vi "Dark_Current_Initialization_Sub_VI.vi"(7 "VISA resource name 2":refnum<visa-resource-name>, 11 "Channel #":i32) -> (0 "error out":errorcluster, 1 "BoardHandle out":T1, 3 "Channel # 2":i32)   [LabVIEW 2018]
uses:
  Program Files (x86)/National Instruments/LabVIEW 2020/instr.lib/CAEN PSM/CAEN PSM.lvlib
panel:
  in  "VISA resource name":refnum<visa-resource-name>
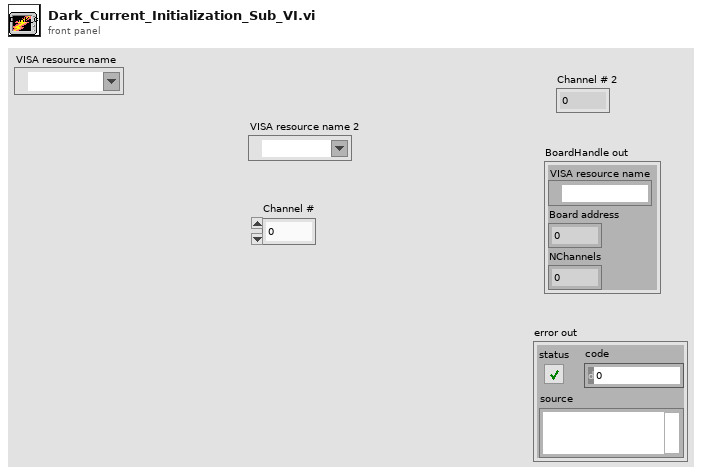
[diagram p1: front panel]
types:
  T1 = cluster{"VISA resource name":refnum<visa-resource-name>, "Board address":u8, "NChannels":u8}
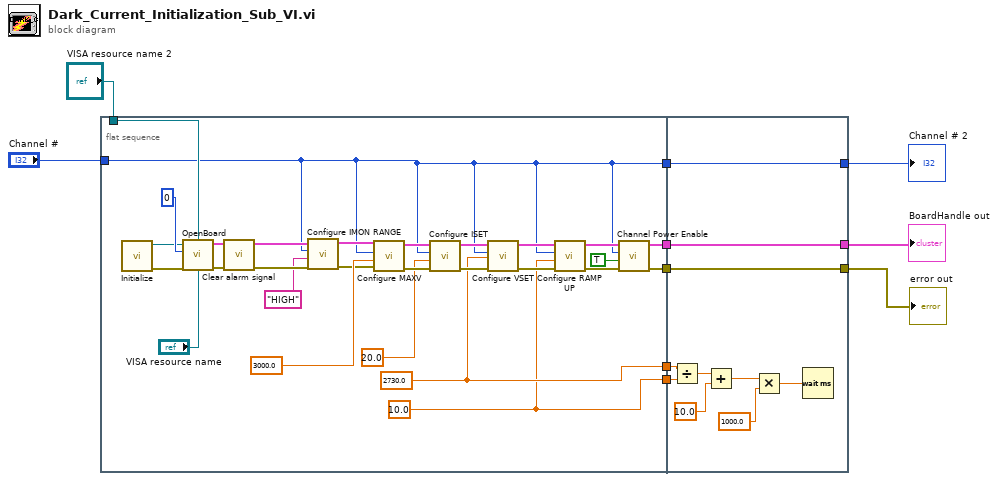
[diagram p0: block diagram]
diagram:
  n1 = flat-sequence {
    tunnel: [w22] -> w10
    tunnel: [w21] -> w9
    tunnel: ["VISA resource name"] -> _
    tunnel: [w20] -> w8
    tunnel: [w19] -> w7
    tunnel: [w11] -> w6
    tunnel: "Channel #" -> [w11]
    tunnel: "VISA resource name 2" -> [_]
    tunnel: w10 -> [w42]
    tunnel: w9 -> [w41]
    tunnel: [w38] -> w3
    tunnel: w8 -> [w38]
    tunnel: [w40] -> w4
    tunnel: w7 -> [w40]
    tunnel: [w39] -> w2
    tunnel: w6 -> [w39]
    frame #0 {
      w22 = 2730.0 ("Voltage Set (Volts)")
      w21 = 10.0 ("Voltage Ramp Up (V/s)")
      n2 = call "Initialize.vi"("VISA resource name"="VISA resource name") -> ("error out"=w32:errorcluster, "VISA resource name out"=w28:refnum<visa-resource-name>)  [unwired: 9 in]
      n3 = call "OpenBoard.vi"("error in (no error)"=w32, "Board Address"=0, "VISA resource name"=w28) -> ("error out"=w33:errorcluster, "BoardHandle"=w27:T1)  [unwired: 7 in]
      n4 = call "Clear alarm signal.vi"("error in (no error)"=w33, "BoardHandle"=w27) -> ("error out"=w17:errorcluster, "BoardHandle out"=w16:T1)  [unwired: 8 in]
      n5 = call "Configure IMON RANGE.vi"("error in (no error)"=w17, "IMon range (LOW)"="HIGH", "Channel (0)"=w11, "BoardHandle"=w16) -> ("error out"=w13:errorcluster, "BoardHandle out"=w14:T1)  [unwired: 6 in]
      n6 = call "Configure MAXV.vi"("error in (no error)"=w13, "Voltage Max (0.0 V)"=3000.0 ("VMax (Volts)"), "Channel (0)"=w11, "BoardHandle"=w14) -> ("error out"=w34:errorcluster, "BoardHandle out"=w26:T1)  [unwired: 6 in]
      n7 = call "Configure ISET.vi"("error in (no error)"=w34, "Current Limit (0.00 uA)"=20.0 ("Current Limit (uA)"), "Channel (0)"=w11, "BoardHandle"=w26) -> ("error out"=w35:errorcluster, "BoardHandle out"=w25:T1)  [unwired: 6 in]
      n8 = call "Configure VSET.vi"("error in (no error)"=w35, "Voltage Level (0.0 V)"=w22, "Channel (0)"=w11, "BoardHandle"=w25) -> ("error out"=w36:errorcluster, "BoardHandle out"=w24:T1)  [unwired: 6 in]
      n9 = call "Configure RAMP UP.vi"("error in (no error)"=w36, "Voltage ramp up (0 V/s)"=w21, "Channel (0)"=w11, "BoardHandle"=w24) -> ("error out"=w37:errorcluster, "BoardHandle out"=w23:T1)  [unwired: 6 in]
      n10 = call "Channel Power Enable.vi"("error in (no error)"=w37, "Enable (OFF)"=TRUE ("Boolean"), "Channel (0)"=w11, "BoardHandle"=w23) -> ("error out"=w19:errorcluster, "BoardHandle out"=w20:T1)  [unwired: 6 in]
    }
    frame #1 {
      n11 = Divide(x=w42, y=w41) -> (x/y=w45:dbl)
      n12 = Add(x=w45, y=10.0) -> (x+y=w46:dbl)
      n13 = Multiply(x=w46, y=1000.0) -> (x*y=w47:dbl)
      n14 = Wait (ms)(milliseconds to wait=w47) -> ()  [unwired: 1 out]
    }
  }
  "error out" <- w4
  "BoardHandle out" <- w3
  "Channel # 2" <- w2
